vi "value_boolean.vi"(5 "operation":T1, 7 "section":string[](array[string]), 8 "error in (no error)":errorcluster, 9 "value in":bool, 10 "key":string[](array[string]), 11 "path in":path) -> (0 "error out":errorcluster, 1 "value out":bool, 2 "exists?":bool, 3 "path out":path)   [LabVIEW 2017, in "toml.lvlib"]
uses:
  toml.lvlib
  value_operation.ctl
  fg_action.ctl
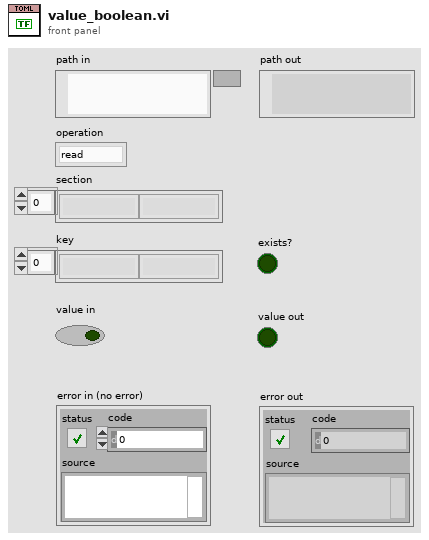
[diagram p1: front panel]
types:
  T1 = typedef "toml.lvlib/value_operation.ctl" = enum8{"read", "write"}
  T2 = typedef "toml.lvlib/fg_action.ctl" = enum8{"null", "get", "set", "pop", "import", "export", "drop", "sections", "keys", "remove"}
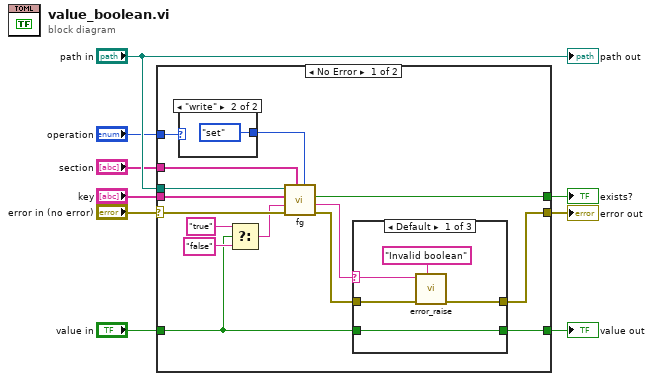
[diagram p0: block diagram]
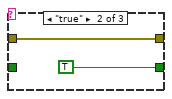
[diagram p2: hidden frame]
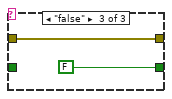
[diagram p3: hidden frame]
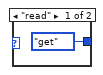
[diagram p4: hidden frame]
diagram:
  n1 = case shown="No Error" "error in (no error)" {
    selector: "error in (no error)" -> [w24 w37]
    tunnel: [w11 w37] -> w8
    tunnel: "path in" -> [w23 _]
    tunnel: "operation" -> [w21 _]
    tunnel: "section" -> [w20 _]
    tunnel: "key" -> [w19 _]
    tunnel: [w18 _] -> w3
    tunnel: [w13 w36] -> w2
    tunnel: "value in" -> [w10 w36]
    frame No Error {
      n2 = case shown="\"write\"" w21 {
        tunnel: [fg_action."get" ("action") fg_action."set" ("action")] -> w22
        frame "read" {
        }
        frame "write" {
        }
      }
      n3 = Select(t="true", s=w10, f="false") -> (s? t:f=w15:string)
      n4 = call "fg.vi"("action"=w22, "section"=w20, "error in (no error)"=w24, "value in"=w15, "key"=w19, "path in"=w23) -> ("error out"=w12:errorcluster, "value out"=w14:string, "exists?"=w18:bool)  [unwired: 2 in, 1 out]
      n5 = case shown="Default" w14 {
        selector: w14 -> [w27 _ _]
        tunnel: [w25 TRUE FALSE] -> w13
        tunnel: [w28 w30 w32] -> w11
        tunnel: w12 -> [w29 w30 w32]
        tunnel: w10 -> [w25 _ _]
        frame Default {
          n6 = call "error_raise.vi"("message"="Invalid boolean", "error in (no error)"=w29, "toml"=w27) -> ("error out"=w28:errorcluster)  [unwired: 8 in]
        }
        frame "true" {
        }
        frame "false" {
        }
      }
    }
    frame Error {
    }
  }
  "error out" <- w8
  "value out" <- w2
  "exists?" <- w3
  "path out" <- "path in"
